vi "Reserve Sessions - N Pins.vi"(6 "timeout (ms)":i32, 8 "error in (no error)":errorcluster, 10 "pin or relay names":string[](array[string]), 11 "measurement context in":refnum<class "MeasurementContext.lvclass">) -> (0 "error out":errorcluster, 2 "session reservation out":refnum<class "Session Reservation.lvclass">, 3 "measurement context out":refnum<class "MeasurementContext.lvclass">)   [LabVIEW 2020, in "MeasurementLink Measurement Server.lvlib" / "MeasurementContext.lvclass"]
doc: "Reserves session(s) based on the provided pin information."
uses:
  MeasurementContext.lvclass
  MeasurementLink Session Management/Session Reservation/Session Reservation.lvclass
  MeasurementContext.lvclass/MeasurementContext.ctl
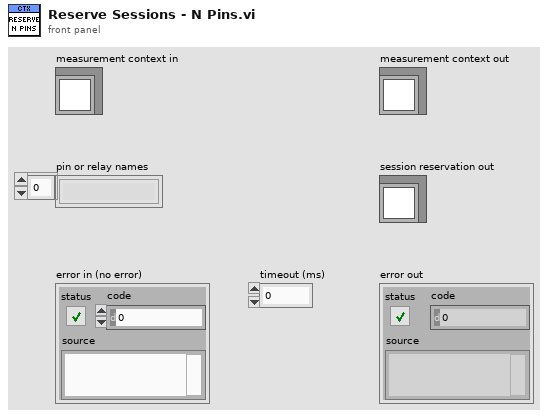
[diagram p1: front panel]
types:
  T1 = typedef "MeasurementLink Measurement Server.lvlib/PinMapContext.ctl" = cluster{"pin_map_id":string, "sites":i32[]}
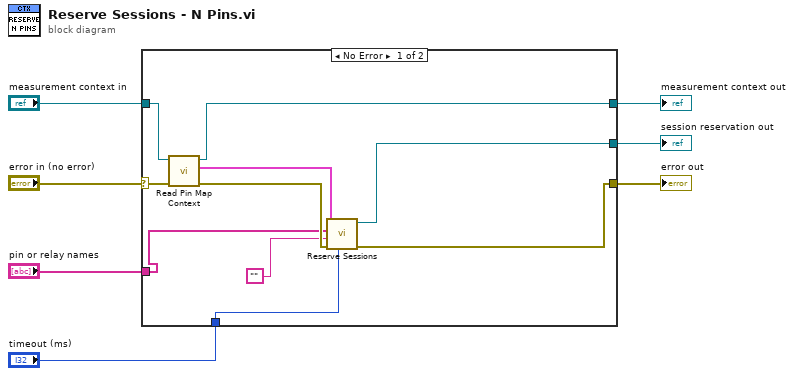
[diagram p0: block diagram]
diagram:
  n1 = case shown="No Error" "error in (no error)" {
    selector: "error in (no error)" -> [w10 w18]
    tunnel: [w17 w18] -> w7
    tunnel: [w16 _] -> w6
    tunnel: "timeout (ms)" -> [w8 _]
    tunnel: "pin or relay names" -> [w13 _]
    tunnel: [w12 w19] -> w3
    tunnel: "measurement context in" -> [w11 w19]
    frame No Error {
      n2 = call-dynamic "Read Pin Map Context.vi"("error in (no error)"=w10, "MeasurementContext in"=w11) -> ("error out"=w14:errorcluster, "pin map context"=w15:T1, "MeasurementContext out"=w12:refnum<class "MeasurementContext.lvclass">)  [unwired: 7 in]
      n3 = call "Reserve Sessions.vi"("timeout (ms)"=w8, "error in (no error)"=w14, "instrument type id"="" ("instrument_type_id"), "pin or relay names"=w13, "pin map context"=w15) -> ("error out"=w17:errorcluster, "session reservation out"=w16:refnum<class "Session Reservation.lvclass">)  [unwired: 5 in]
    }
    frame Error {
    }
  }
  "error out" <- w7
  "session reservation out" <- w6
  "measurement context out" <- w3
